vi "NPI_Control.vi"(8 "error in (no error)":errorcluster, 9 "Color Box":u32(colorbox), 10 "No. NeoPixel":u8=1 max=2, 11 "VISA resource name":refnum<visa-resource-name>) -> (0 "error out":errorcluster, 3 "VISA resource name out":refnum<visa-resource-name>)   [LabVIEW 2025]
doc: "Este VI permite controlar individualmente la NeoPixel seleccionada de 0 a 2 de la placa Galiot \nSe debe indicar que neopixel se usara y que color se elegira"
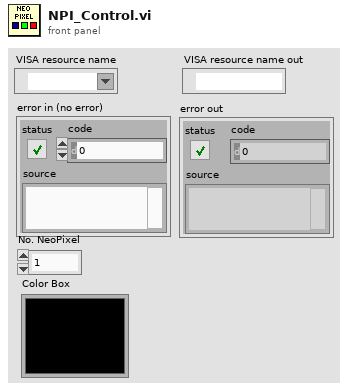
[diagram p1: front panel]
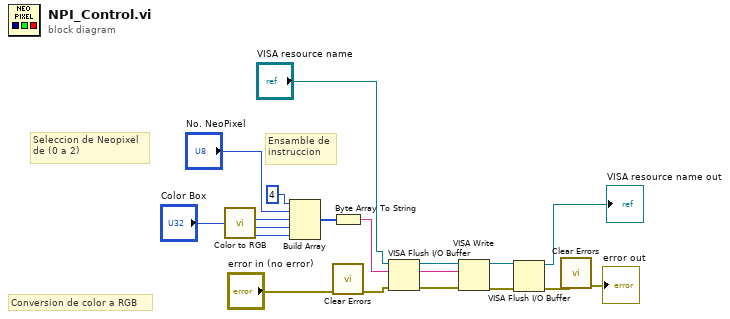
[diagram p0: block diagram]
diagram:
  # "Ensamble de\ninstruccion"
  # "Conversion de color a RGB"
  # "Seleccion de Neopixel\nde (0 a 2)"
  n1 = call <vilib>:"Color to RGB.vi"("Color"="Color Box") -> ("R"=w16:u8, "G"=w15:u8, "B"=w14:u8)  [unwired: 1 out]
  n2 = Build Array(u8 4 ("element"), "No. NeoPixel", w16, w15, w14) -> (w13:u8[])
  n3 = Byte Array To String(unsigned byte array=w13) -> (string=w18:string)
  n4 = call <vilib>:"Clear Errors.vi"("error in (no error)"="error in (no error)") -> ("error out"=w1:errorcluster)  [unwired: 5 in, 1 out]
  n5 = VISA Flush I/O Buffer(VISA resource name="VISA resource name", error in (no error)=w1) -> (VISA resource name out=w3:refnum<visa-resource-name>, error out=w4:errorcluster)  [unwired: 1 in]
  n6 = VISA Write(VISA resource name=w3, write buffer=w18, error in (no error)=w4) -> (VISA resource name out=w6:refnum<visa-resource-name>, error out=w7:errorcluster)  [unwired: 1 out]
  n7 = VISA Flush I/O Buffer(VISA resource name=w6, error in (no error)=w7) -> (VISA resource name out=→"VISA resource name out":refnum<visa-resource-name>, error out=w8:errorcluster)  [unwired: 1 in]
  n8 = call <vilib>:"Clear Errors.vi"("error in (no error)"=w8) -> ("error out"=→"error out":errorcluster)  [unwired: 5 in, 1 out]
